vi "Solve Linear Equations.vi"   [LabVIEW 2020, in "NI_AALPro.lvlib"]
doc: "Solves a linear system AX = Y. The data types you wire to the <B>Input Matrix</B> and <B>Known Vector</B> inputs determine the polymorphic instance to use."
uses:
  <vilib>/Analysis/NI_AALPro.lvlib
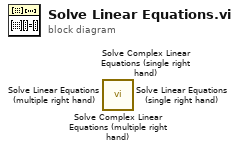
[diagram p0: block diagram]
diagram:
  n1 = call <vilib>:"Solve Complex Linear Equations (multiple right hand).vi"() -> ()  [unwired: 3 in, 2 out]
  n2 = call <vilib>:"Solve Complex Linear Equations (single right hand).vi"() -> ()  [unwired: 3 in, 2 out]
  n3 = call <vilib>:"Solve Linear Equations (multiple right hand).vi"() -> ()  [unwired: 3 in, 2 out]
  n4 = call <vilib>:"Solve Linear Equations (single right hand).vi"() -> ()  [unwired: 3 in, 2 out]
